vi "MainPanel_20170525.vi"() -> (0 "ErrorOut":errorcluster)   [LabVIEW 2018] (continued)
  # "Cluster data flow is predominantly top to bottom with data being passed using queues.  The Event Structure drives the Main (Consumer) Loop which acts as the Supervisor or dominant loop in this architecture.  In doing so, it handles the functionality of the other loops in your program.  The Consumer Loop processes the 'event' and then if necessary, sends the Master Cluster or a sub-cluster by means of a queue down to the Hardware Loop.  The Hardware loop checks the queued event's data for new information and if there is none, uses the previous iteration's cluster from the Shift Register.  Depending on the mode/event of the Hardware loop, the Hardware Loop may need to update the Master Cluster and does so by pushing the Refresh Panel Queue event which passes the cluster up to the Consumer loop for processing and panel update.  Note that there is a Functional Global inside of the UpdateMasterCluster.vi that is used to maintain a copy of the Master Cluster in memory that can be accessed from anywhere in the software (subVIs included).  This is not always and is often quite unnecessary, but is shown to illustrate a way of passing data between loops without using a Queue.  This use of a FG is quite effective, but must be used with care in that you need to be cautious with where and how often you update the FG; too many writers can cause unpredictable and very challenging code to debug.  The Functional Global exists to allow for any point anywhere in the program and in any loop to grab a copy of your cluster.  This architecture is intended to be a solid starting point for most applications, but you will need to configure and tailor the framework for your specific application and the use of some of the concepts shown herein cannot and should not always be used precisely as shown or at all.\n\nGeneral Rules:\n\n- Don't touch your Hardware anywhere except the HW loop.\n- Try to dedicate loops to very specific tasks to compartmentalize your code as much as possible as this helps with readability and scalability.\n- Any and all periodic updates (logging to disk, graph updates to name two) should occur only in the GUI loop.  Periodic updates of front panel indicators in any other loop will cause unnecessary loop cycles.\n- State changes for the program (ie. Idle, Run, Stop, Error) are handled in the Main Loop only and the panel is updated accordingly. \n- Use the Refresh Panel case in the Main Loop to handle all state changes and Panel GUI configuration tasks (enable/disable controls, visible, colors, alarming, status indicators, etc.).\n- Most loops only run when called by event/queue at the prescribed rate of the software.  Depending on your application, timed or free-wheeling loops could be implemented here if desired, but free-wheeling loops can be inefficient if not carefully implemented.\n- There are a couple of cases such as InitSW that are currently only called upon initialization and never again as shown below and one could argue that they could be outside of the architecture, but if they are called once, they may need to be again, so it is helpful to include them in the overall architecture for potential future use.  An example of this would be InitHW as in the event of a HW failure resulting from poor configuration choices, it would be helpful to be able to call the InitHW case again to reinitialize the HW with new settings."
  n1 = Current VI's Path() -> (path=w82:path)
  n2 = Current VI's Path() -> (path=w88:path)
  n3 = Strip Path(path=w82) -> (stripped path=w81:path)  [unwired: 1 out]
  n4 = Strip Path(path=w88) -> (stripped path=w87:path)  [unwired: 1 out]
  n5 = Strip Path(path=w81) -> (stripped path=w80:path)  [unwired: 1 out]
  n6 = Current VI's Path() -> (path=w98:path)
  n7 = Current VI's Path() -> (path=w90:path)
  n8 = Strip Path(path=w87) -> (stripped path=w86:path)  [unwired: 1 out]
  n9 = Strip Path(path=w98) -> (stripped path=w97:path)  [unwired: 1 out]
  n10 = Strip Path(path=w90) -> (stripped path=w91:path)  [unwired: 1 out]
  n11 = flat-sequence {
    tunnel: [w172] -> w115
    tunnel: errorcluster {"status"=FALSE, "code"=0, "source"=""} ("ErrorIn") -> [w171]
    frame #0 {
      w169 = -1 ("FAM Init 1")
      n12 = shared-variable ".\\Connex_Variables.lvlib\\10Hz_File_Refs"(T45 {"72Co_dset"=0, "84Co_dset"=0, "FileRef"=0} ("10Hz_File_Refs"), error in=w171) -> (error out=w172:errorcluster)
      n13 = shared-variable ".\\Connex_Variables.lvlib\\FAM Init 2"(w169) -> ()  [unwired: 1 in, 1 out]
      n14 = shared-variable ".\\Connex_Variables.lvlib\\FAM Init 1"(w169) -> ()  [unwired: 1 in, 1 out]
      n15 = shared-variable ".\\Connex_Variables.lvlib\\TCP_Status"(TRUE ("TCP_Status")) -> ()  [unwired: 1 in, 1 out]
      n16 = local write "Exit"(FALSE ("Exit")) -> ()
    }
  }
  n17 = Strip Path(path=w97) -> (stripped path=w96:path)  [unwired: 1 out]
  n18 = Strip Path(path=w91) -> (stripped path=w92:path)  [unwired: 1 out]
  n19 = Build Path(base path=w86, name or relative path="NASA\\wtle_young_weather_stn\\WeatherStationMain_20180517.vi") -> (appended path=w84:path)
  n20 = Build Path(base path=w80, name or relative path="NASA\\statmon_2015\\ADAM_health_subpanel_20190329.vi") -> (appended path=w78:path)
  n21 = Obtain Queue(max queue size (-1, unlimited)=100, name (unnamed)="Supervisor", element data type=w165, error in (no error)=w115) -> (queue out=w166:refnum<queue>, error out=w167:errorcluster)  [unwired: 1 in, 1 out]
  n22 = Build Path(base path=w96, name or relative path="Disdrometer\\disdrometer_2020_09_09.vi") -> (appended path=w94:path)
  n23 = Build Path(base path=w92, name or relative path="NASA\\te_2015\\te_20200903.vi") -> (appended path=w89:path)
  n24 = Enqueue Element(queue=w166, element=w165, error in (no error)=w167) -> (queue out=w148:refnum<queue>, error out=w1:errorcluster)  [unwired: 2 out]
  n25 = Open VI Reference(vi path=w78, error in (no error)=w1) -> (vi reference=w74:refnum<vi>, error out=w42:errorcluster)  [unwired: 4 in]
  n26 = Open VI Reference(vi path=w94, error in (no error)=w1) -> (vi reference=w73:refnum<vi>, error out=w57:errorcluster)  [unwired: 4 in]
  n27 = Open VI Reference(vi path=w89, error in (no error)=w1) -> (vi reference=w72:refnum<vi>, error out=w40:errorcluster)  [unwired: 4 in]
  n28 = Open VI Reference(vi path=w84, error in (no error)=w1) -> (vi reference=w16:refnum<vi>, error out=w28:errorcluster)  [unwired: 4 in]
  n29 = invoke on="DisdroPanel" class="SubPnl" method="Insert VI"(error in=w57, "VI Ref"=w73) -> (error out=w54:errorcluster)  [unwired: 2 in, 3 out]
  n30 = invoke on="TE_panel" class="SubPnl" method="Insert VI"(error in=w40, "VI Ref"=w72) -> (error out=w30:errorcluster)  [unwired: 2 in, 3 out]
  n31 = invoke on="Sub Panel - Weather" class="SubPnl" method="Insert VI"(error in=w28, "VI Ref"=w16) -> (error out=w18:errorcluster)  [unwired: 2 in, 3 out]
  n32 = Obtain Queue(max queue size (-1, unlimited)=100, name (unnamed)="Data", element data type=w122, error in (no error)=w1) -> (queue out=w126:refnum<queue>, error out=w124:errorcluster)  [unwired: 1 in, 1 out]
  n33 = Obtain Queue(max queue size (-1, unlimited)=110, name (unnamed)="FP", element data type=w99, error in (no error)=w1) -> (queue out=w102:refnum<queue>, error out=w101:errorcluster)  [unwired: 1 in, 1 out]
  n34 = invoke on="ADAM Health" class="SubPnl" method="Insert VI"(error in=w42, "VI Ref"=w74) -> (error out=w41:errorcluster)  [unwired: 2 in, 3 out]
  n35 = Obtain Queue(max queue size (-1, unlimited)=100, name (unnamed)=w119, element data type=cluster{"HWMd":T25, "Data":variant} {"HWMd"=enum."HW_Init", "Data"=variant}, error in (no error)=w1) -> (queue out=w154:refnum<queue>, error out=w153:errorcluster)  [unwired: 1 in, 1 out]
  n36 = Obtain Queue(max queue size (-1, unlimited)=100, name (unnamed)=w118, element data type=cluster{"HWMd":T25, "Data":variant} {"HWMd"=enum."HW_Init", "Data"=variant}, error in (no error)=w1) -> (queue out=w65:refnum<queue>, error out=w135:errorcluster)  [unwired: 1 in, 1 out]
  n37 = Enqueue Element(queue=w126, element=w122, error in (no error)=w124) -> (queue out=w125:refnum<queue>, error out=w123:errorcluster)  [unwired: 1 in, 1 out]
  n38 = Obtain Queue(max queue size (-1, unlimited)=100, name (unnamed)="10Hz", element data type=cluster{"Enum":T19, "Var":variant} {"Enum"=enum."10Hz_Init", "Var"=variant}) -> (queue out=w14:refnum<queue>, error out=w15:errorcluster)  [unwired: 2 in, 1 out]
  n39 = Obtain Queue(max queue size (-1, unlimited)=1000, name (unnamed)="Tones", element data type=cluster{"Enum":T43, "Data":variant} {"Enum"=enum."Data_Init", "Data"=variant}, error in (no error)=w1) -> (queue out=w149:refnum<queue>, error out=w160:errorcluster)  [unwired: 1 in, 1 out]
  n40 = Obtain Queue(max queue size (-1, unlimited)=100, name (unnamed)="Digi", element data type=w128, error in (no error)=w1) -> (queue out=w132:refnum<queue>, error out=w130:errorcluster)  [unwired: 1 in, 1 out]
  n41 = Obtain Queue(max queue size (-1, unlimited)=100, name (unnamed)="Log", element data type=w4, error in (no error)=w1) -> (queue out=w5:refnum<queue>, error out=w76:errorcluster)  [unwired: 1 in, 1 out]
  n42 = Obtain Queue(max queue size (-1, unlimited)=100, name (unnamed)="TCP", element data type=w7) -> (queue out=w11:refnum<queue>)  [unwired: 2 in, 2 out]
  n43 = Enqueue Element(queue=w102, element=w99, error in (no error)=w101) -> (queue out=w77:refnum<queue>, error out=w100:errorcluster)  [unwired: 1 in, 1 out]
  n44 = Enqueue Element(queue=w5, element=w4, error in (no error)=w76) -> (queue out=w6:refnum<queue>, error out=w12:errorcluster)  [unwired: 1 in, 1 out]
  n45 = Enqueue Element(queue=w11, element=w7) -> (queue out=w2:refnum<queue>, error out=w8:errorcluster)  [unwired: 2 in, 1 out]
  n46 = invoke class="VI" method="Run VI"(reference=w16, error in=w18, "Wait until done"=FALSE ("Wait Until Done"), "Auto Dispose Ref"=FALSE ("Auto Dispose Reference")) -> (error out=w17:errorcluster)  [unwired: 1 in, 4 out]
  n47 = invoke class="VI" method="Run VI"(reference=w74, error in=w41, "Wait until done"=FALSE ("Wait Until Done"), "Auto Dispose Ref"=FALSE ("Auto Dispose Reference")) -> (error out=w43:errorcluster)  [unwired: 1 in, 4 out]
  n48 = invoke class="VI" method="Run VI"(reference=w73, error in=w54, "Wait until done"=FALSE ("Wait Until Done"), "Auto Dispose Ref"=FALSE ("Auto Dispose Reference")) -> (error out=w53:errorcluster)  [unwired: 1 in, 4 out]
  n49 = invoke class="VI" method="Run VI"(reference=w72, error in=w30, "Wait until done"=FALSE ("Wait Until Done"), "Auto Dispose Ref"=FALSE ("Auto Dispose Reference")) -> (error out=w29:errorcluster)  [unwired: 1 in, 4 out]
  n50 = Enqueue Element(queue=w132, element=w128, error in (no error)=w130) -> (queue out=w131:refnum<queue>, error out=w129:errorcluster)  [unwired: 1 in, 1 out]
  n51 = call "NoiseLoop.vi"("error in (no error)"=w123, "Queue in"=w125) -> ("error out"=w147:errorcluster)  [unwired: 9 in]
  n52 = call "LogLoop_HDF5_20190307.vi"("error in"=w12, "Queue in"=w6) -> ("error out"=w109:errorcluster)  [unwired: 9 in]
  n53 = call "Simple TCP - Server_20211123.vi"("error in"=w8, "TCP_Q"=w2) -> ("error out"=w3:errorcluster)  [unwired: 8 in, 1 out]
  n54 = call "DigitalOutput.vi"("error in (no error)"=w129, "Queue in"=w131) -> ("error out"=w120:errorcluster)  [unwired: 9 in]
  n55 = call "10HzLogLoop_HDF5_20210610.vi"("error in"=w15, "queue in"=w14) -> ("error out"=w66:errorcluster)  [unwired: 9 in]
  n56 = while {
    tunnel: w1 -> [w177]
    tunnel: [w175] -> w106
    stop <- w180 stop-if-true
    n57 = call "Elapsed Time"("Time Target (s)"="MemoryPlotRate") -> ("Time has Elapsed"=w179:bool)  [unwired: 11 in, 7 out]
    n58 = Wait Until Next ms Multiple(millisecond multiple=u32 50) -> ()  [unwired: 1 out]
    n59 = case shown="True" w179 {
      tunnel: w177 -> [w181 w184]
      tunnel: [w181 w182] -> w175
      frame False {
      }
      frame True {
        # "When we were using the watchdog to reset Windows,\nwe were checking here. Now that we're only using it to\nnotify WSCR, we're doing it in Log_SSH."
        n60 = constructor class="Process"(error in=w184) -> (reference out=w194:refnum<k24>, error out=w185:errorcluster)  [unwired: 2 in, 1 out]
        n61 = invoke class="Process" method="GetCurrentProcess"(reference=w194, error in=w185) -> (reference out=w192:refnum<k24>, error out=w193:errorcluster, "GetCurrentProcess"=w186:refnum<k24>)  [unwired: 1 in]
        n62 = property class="Process"(reference=w186, error in=w193) -> (reference out=w190:refnum<k24>, error out=w189:errorcluster, "WorkingSet"=w187:i32)
        n63 = Divide(x=w187, y=i64 1024) -> (x/y=→"Memory Used By LV (KB)" →"Memory Used":dbl)
        n64 = Close Reference(reference=w190, error in (no error)=w189) -> (error out=w191:errorcluster)
        n65 = Close Reference(reference=w192, error in (no error)=w191) -> (error out=w182:errorcluster)
      }
    }
    n66 = local read "Exit"() -> (w180:bool)
  }
  n67 = call "TonesLoop_20190705.vi"("WeightOfNewFrequency"=1.0, "error in"=w160, "Queue in"=w149) -> ("error out"=w150:errorcluster)  [unwired: 8 in]
  n68 = while {
    tunnel: w148 -> [w198]
    shift-right: [w197] -> w159
    shift-left: w1 -> [w199]
    stop <- w196 stop-if-true
    n69 = event shown="[7] \"base path\", \"NAS path\", \"ThreshFile\", \"Location\": Value Change" {
      selector: _ -> [_ _ _ _ _ _ _ _ _ _ _ _ _ _]
      dyn-events: _ -> [_ _ _ _ _ _ _ _ _ _ _ _ _ _]
      timeout: 100 -> [_ _ _ _ _ _ _ _ _ _ _ _ _ _]
      tunnel: w199 -> [w204 w208 w221 w227 w229 w233 w241 w249 w257 w260 w265 w269 w273 w277]
      tunnel: w198 -> [_ w215 w216 w222 w230 w234 w242 w250 w258 w262 w266 w270 w274 w279]
      tunnel: [w204 w207 w217 w223 w228 w232 w240 w248 w256 w261 w264 w268 w275 w278] -> w197
      tunnel: [_ w206 _ _ _ _ _ _ _ _ _ _ _ TRUE] -> w196
      event Timeout {
        # "13:24:24.3\n05/31/2018"
        # "Timeout Case is used to update 'heartbeat' clock on the front panel to provide an indication that the software is still running"
        n70 = event-data() -> ()  [unwired: 2 out]
        n71 = Get Date/Time In Seconds() -> (seconds since 1Jan1904=w203:timestamp)
        n72 = Format Date/Time String(time format string (%c)="%H:%M:%S%1u\n%m/%d/%Y", seconds (now)=w203, UTC format=TRUE) -> (date/time string=→"UTC date/time":string)
      }
      event Menu Selection (User) {
        # "This handles a menu selection while the program is running."
        n73 = event-data() -> ("ItemTag"=w209:string)  [unwired: 1 out]
        n74 = Scan From String(input string=w209, error in=w208, default 1=MainQueueElements."Spvsr_InitQ" ("QElmnt")) -> (error out=w205:errorcluster, output 1=w213:T44)  [unwired: 2 in, 2 out]
        n75 = Bundle(cluster=cluster{"QElmnt":T44, "Data":variant} {"QElmnt"=enum."Spvsr_InitQ", "Data"=variant} ("Cluster"), "QElmnt"=w213) -> (w212:cluster{"QElmnt":T44, "Data":variant})  [unwired: 1 in]
        n76 = Enqueue Element(queue=w215, element=w212, error in (no error)=w205) -> (error out=w207:errorcluster)  [unwired: 3 out]
        n77 = Equal?(x=MainQueueElements."Spvsr_Exit" ("QElmnt"), y=w213) -> (x = y?=w206:bool)
      }
      event "Config": Value Change {
        n78 = event-data() -> ()  [unwired: 2 out]
        n79 = Enqueue Element(queue=w216, element=cluster{"QElmnt":T44, "Data":variant} {"QElmnt"=enum."Spvsr_Config", "Data"=variant} ("Cluster"), error in (no error)=w221) -> (error out=w218:errorcluster)  [unwired: 3 out]
        n80 = Enqueue Element(queue=w216, element=cluster{"QElmnt":T44, "Data":variant} {"QElmnt"=enum."Spvsr_FPConfig", "Data"=variant} ("Cluster"), error in (no error)=w218) -> (error out=w217:errorcluster)  [unwired: 3 out]
      }
      event "AutoOffset": Value Change {
        n81 = event-data() -> ()  [unwired: 2 out]
        n82 = Enqueue Element(queue=w222, element=cluster{"QElmnt":T44, "Data":variant} {"QElmnt"=enum."Spvsr_DigitzOffs", "Data"=variant} ("Cluster"), error in (no error)=w227) -> (error out=w224:errorcluster)  [unwired: 3 out]
        n83 = Enqueue Element(queue=w222, element=cluster{"QElmnt":T44, "Data":variant} {"QElmnt"=enum."Spvsr_FPConfig", "Data"=variant} ("Cluster"), error in (no error)=w224) -> (error out=w223:errorcluster)  [unwired: 3 out]
      }
      event "FreqsToRemove", "AvgAvg", "SNR_Thresh", "Width [bins]", "FreqsToRemove 2", "Width 2 [bins]", "SimulateFPGA": Value Change {
        n84 = event-data() -> ()  [unwired: 2 out]
        n85 = Enqueue Element(queue=w230, element=cluster{"QElmnt":T44, "Data":variant} {"QElmnt"=enum."Spvsr_FPConfig", "Data"=variant} ("Cluster"), error in (no error)=w229) -> (error out=w228:errorcluster)  [unwired: 3 out]
      }
      event "MaxTrackRate": Value Change {
        n86 = event-data() -> ()  [unwired: 6 out]
        n87 = for {
          tunnel: cluster{"QElmnt":T44, "Data":variant}[] [{"QElmnt"=enum."Spvsr_FPConfig", "Data"=variant}, {"QElmnt"=enum."Spvsr_TrackRate", "Data"=variant}] ("Cluster") -> [w238] mode=indexing
          tunnel: w234 -> [w237]
          shift-right: [w236] -> w232
          shift-left: w233 -> [w239]
          n88 = Enqueue Element(queue=w237, element=w238, error in (no error)=w239) -> (error out=w236:errorcluster)  [unwired: 3 out]
        }
      }
      event "AutoCenter": Value Change {
        n89 = event-data() -> ()  [unwired: 6 out]
        n90 = for {
          tunnel: cluster{"QElmnt":T44, "Data":variant}[] [{"QElmnt"=enum."Spvsr_FPConfig", "Data"=variant}, {"QElmnt"=enum."Spvsr_AutoCenter", "Data"=variant}] ("Cluster") -> [w246] mode=indexing
          tunnel: w242 -> [w245]
          shift-right: [w244] -> w240
          shift-left: w241 -> [w247]
          n91 = Enqueue Element(queue=w245, element=w246, error in (no error)=w247) -> (error out=w244:errorcluster)  [unwired: 3 out]
        }
      }
      event "base path", "NAS path", "ThreshFile", "Location": Value Change {
        n92 = event-data() -> ()  [unwired: 6 out]
        n93 = for {
          tunnel: cluster{"QElmnt":T44, "Data":variant}[] [{"QElmnt"=enum."Spvsr_FPConfig", "Data"=variant}, {"QElmnt"=enum."Spvsr_RestartWarn", "Data"=variant}] ("Cluster") -> [w254] mode=indexing
          tunnel: w250 -> [w253]
          shift-right: [w252] -> w248
          shift-left: w249 -> [w255]
          n94 = Enqueue Element(queue=w253, element=w254, error in (no error)=w255) -> (error out=w252:errorcluster)  [unwired: 3 out]
        }
      }
      event "Beacon", "Beacon 3": Cursor Move {
        n95 = event-data() -> ()  [unwired: 2 out]
        n96 = Enqueue Element(queue=w258, element=cluster{"QElmnt":T44, "Data":variant} {"QElmnt"=enum."Spvsr_Cursors", "Data"=variant} ("Cluster"), error in (no error)=w257) -> (error out=w256:errorcluster)  [unwired: 3 out]
      }
      event "noise_ctrl", "72GHz_ctrl", "84GHz_ctrl": Value Change {
        n97 = event-data() -> ()  [unwired: 6 out]
        n98 = Enqueue Element(queue=w262, element=cluster{"QElmnt":T44, "Data":variant} {"QElmnt"=enum."FP_AO_ctrl", "Data"=variant} ("Cluster"), error in (no error)=w260) -> (error out=w261:errorcluster)  [unwired: 3 out]
      }
      event "Zoom On Peak", "AutoScale Y Noise", "AutoScale Y Tones": Value Change {
        n99 = event-data() -> ()  [unwired: 2 out]
        n100 = Enqueue Element(queue=w266, element=cluster{"QElmnt":T44, "Data":variant} {"QElmnt"=enum."Spvsr_FPConfig", "Data"=variant} ("Cluster"), error in (no error)=w265) -> (error out=w264:errorcluster)  [unwired: 3 out]
      }
      event Value Change; Key Up {
        n101 = event-data() -> ()  [unwired: 5 out]
        n102 = Enqueue Element(queue=w270, element=cluster{"QElmnt":T44, "Data":variant} {"QElmnt"=enum."Spvsr_AlarmCfg", "Data"=variant} ("Cluster"), error in (no error)=w269) -> (error out=w268:errorcluster)  [unwired: 3 out]
      }
      event "Stop": Value Change {
        n103 = event-data() -> ()  [unwired: 2 out]
        n104 = Enqueue Element(queue=w274, element=cluster{"QElmnt":T44, "Data":variant} {"QElmnt"=enum."Spvsr_Stop", "Data"=variant} ("Cluster"), error in (no error)=w273) -> (error out=w275:errorcluster)  [unwired: 3 out]
      }
      event "Exit": Value Change; Panel Close {
        n105 = event-data() -> ()  [unwired: 2 out]
        n106 = Enqueue Element(queue=w279, element=cluster{"QElmnt":T44, "Data":variant} {"QElmnt"=enum."Spvsr_Exit", "Data"=variant} ("Cluster"), error in (no error)=w277) -> (error out=w278:errorcluster)  [unwired: 3 out]
      }
    }
  }
  n107 = call "AI_Loop.vi"("error in"=w1, "AI_Type"=AI_Type_Enum."AI") -> ("error out"=w121:errorcluster)  [unwired: 9 in]
  n108 = call "AI_Loop.vi"("error in"=w1, "AI_Type"=AI_Type_Enum."TC") -> ("error out"=w112:errorcluster)  [unwired: 9 in]
  n109 = call "AO_Loop.vi"("error"=w1) -> ("error out"=w110:errorcluster)  [unwired: 10 in]
  n110 = while {
    shift-right: [w294] -> w158
    shift-left: w1 -> [w293]
    tunnel: w148 -> [w284]
    shift-right: [w295] -> _
    shift-left: T29 {"Admin"={"Lvl"=enum."Admin", "Pwd"=""}, "RTConfig"={"Arm"=FALSE, "Number"=0.0, "String"=""}, "SMS"={"Enbl?"=FALSE, "Addr"=[]}, "FPGA"={"Target"=enum."1", "Channel"=enum."1", "Ref1"=refnum, "Ref2"=refnum}, "Config"={"UsrCfg"={"Paths"={"CfgFile"=path "", "LogFolder"=path "", "LogFile"=path "", "NAS path"=path "", "ThreshFile"=path "", "RedunFolder"=path ""}, "SampleRate"=0.0}, "FP_User"={"#NoiseSums"=0, "Max_df"=0, "AvgAvg"=FALSE, "#Avg"=0, "AutoCenter"=FALSE, "Inclin"={"Vmin"=0.0, "Vmax"=0.0, "Angle_min"=0.0, "Angle_max"=0.0, "Offset"=0.0, "Pos_Neg"=FALSE}, "1"={"Cal_"={"Fine"=0.0, "Coarse_"=0.0}, "Beac"={"Fine"=0.0, "Coarse_"=0.0}, "Scale"={"Step4"=0.0, "Step5"=0.0, "Step6"=0.0, "Step7"=0.0}, "Offset"=0.0, "Scale_Noise"=0.0, "Scale_Step1"=0.0, "Scale_In_RT"=0.0, "ScaleMeas"=0.0, "FreqsToRemove"=[], "Width"=[], "ScaleMeasEnum"=enum."1", "FilterEnab"=enum."None"}, "2"={"Cal_"={"Fine"=0.0, "Coarse_"=0.0}, "Beac"={"Fine"=0.0, "Coarse_"=0.0}, "Scale"={"Step4"=0.0, "Step5"=0.0, "Step6"=0.0, "Step7"=0.0}, "Offset"=0.0, "Scale_Noise"=0.0, "Scale_Step1"=0.0, "Scale_In_RT"=0.0, "ScaleMeas"=0.0, "FreqsToRemove"=[], "Width"=[], "ScaleMeasEnum"=enum."1", "FilterEnab"=enum."None"}, "3"={"Cal_"={"Fine"=0.0, "Coarse_"=0.0}, "Beac"={"Fine"=0.0, "Coarse_"=0.0}, "Scale"={"Step4"=0.0, "Step5"=0.0, "Step6"=0.0, "Step7"=0.0}, "Offset"=0.0, "Scale_Noise"=0.0, "Scale_Step1"=0.0, "Scale_In_RT"=0.0, "ScaleMeas"=0.0, "FreqsToRemove"=[], "Width"=[], "ScaleMeasEnum"=enum."1", "FilterEnab"=enum."None"}, "4"={"Cal_"={"Fine"=0.0, "Coarse_"=0.0}, "Beac"={"Fine"=0.0, "Coarse_"=0.0}, "Scale"={"Step4"=0.0, "Step5"=0.0, "Step6"=0.0, "Step7"=0.0}, "Offset"=0.0, "Scale_Noise"=0.0, "Scale_Step1"=0.0, "Scale_In_RT"=0.0, "ScaleMeas"=0.0, "FreqsToRemove"=[], "Width"=[], "ScaleMeasEnum"=enum."1", "FilterEnab"=enum."None"}, "Target to Probe"=enum."1", "SNR_Thresh"=0.0, "Paths"={"CfgFile"=path "", "LogFolder"=path "", "LogFile"=path "", "NAS path"=path "", "ThreshFile"=path "", "RedunFolder"=path ""}, "Connex_Location"="", "SimulateFPGA"=FALSE, "Deadband"=0.0}}, "Stat"={"SysState"=enum."Init", "TrackRate"=FALSE, "AutoCentr"=FALSE}, "Alarm"={"TC13"={"Enbl"=FALSE, "ErrsAndWarns"={0.0, 0.0, 0.0, 0.0}}, "AI1"={"Enbl"=FALSE, "ErrsAndWarns"={0.0, 0.0, 0.0, 0.0}}, "AI2"={"Enbl"=FALSE, "ErrsAndWarns"={0.0, 0.0, 0.0, 0.0}}, "AI3"={"Enbl"=FALSE, "ErrsAndWarns"={0.0, 0.0, 0.0, 0.0}}, "AI4"={"Enbl"=FALSE, "ErrsAndWarns"={0.0, 0.0, 0.0, 0.0}}, "AI5"={"Enbl"=FALSE, "ErrsAndWarns"={0.0, 0.0, 0.0, 0.0}}, "AI6"={"Enbl"=FALSE, "ErrsAndWarns"={0.0, 0.0, 0.0, 0.0}}, "AI18"={"Enbl"=FALSE, "ErrsAndWarns"={0.0, 0.0, 0.0, 0.0}}, "AI19"={"Enbl"=FALSE, "ErrsAndWarns"={0.0, 0.0, 0.0, 0.0}}, "TE1"={"Enbl"=FALSE, "ErrsAndWarns"={0.0, 0.0, 0.0, 0.0}}, "TE2"={"Enbl"=FALSE, "ErrsAndWarns"={0.0, 0.0, 0.0, 0.0}}, "TE3"={"Enbl"=FALSE, "ErrsAndWarns"={0.0, 0.0, 0.0, 0.0}}, "ADAM1"={"Enbl"=FALSE, "ErrsAndWarns"={0.0, 0.0, 0.0, 0.0}}, "ADAM2"={"Enbl"=FALSE, "ErrsAndWarns"={0.0, 0.0, 0.0, 0.0}}, "ADAM3"={"Enbl"=FALSE, "ErrsAndWarns"={0.0, 0.0, 0.0, 0.0}}, "ADAM4"={"Enbl"=FALSE, "ErrsAndWarns"={0.0, 0.0, 0.0, 0.0}}, "72CoBeacFreq"={"Enbl"=FALSE, "ErrsAndWarns"={0.0, 0.0, 0.0, 0.0}}, "72CoCalFreq"={"Enbl"=FALSE, "ErrsAndWarns"={0.0, 0.0, 0.0, 0.0}}, "84CoBeacFreq"={"Enbl"=FALSE, "ErrsAndWarns"={0.0, 0.0, 0.0, 0.0}}, "84CoCalFreq"={"Enbl"=FALSE, "ErrsAndWarns"={0.0, 0.0, 0.0, 0.0}}, "72Co_CalTonePwr"={"Enbl"=FALSE, "ErrsAndWarns"={0.0, 0.0, 0.0, 0.0}}, "72X_CalTonePwr"={"Enbl"=FALSE, "ErrsAndWarns"={0.0, 0.0, 0.0, 0.0}}, "84Co_CalTonePwr"={"Enbl"=FALSE, "ErrsAndWarns"={0.0, 0.0, 0.0, 0.0}}, "84X_CalTonePwr"={"Enbl"=FALSE, "ErrsAndWarns"={0.0, 0.0, 0.0, 0.0}}}} ("ClusterIn") -> [w302]
    tunnel: w154 -> [w290]
    tunnel: w149 -> [w289]
    tunnel: w125 -> [w288]
    tunnel: w6 -> [w287]
    tunnel: w77 -> [w286]
    tunnel: w14 -> [w282]
    tunnel: w65 -> [w281]
    i -> [w285]
    stop <- w301 stop-if-true
    # "MasterCluster"
    # "Main \n(Supervisor)\nLoop"
    # "Supervisor Loop"
    n111 = call "PushToErrorHandler.vi"("ErrorIn"=w293, "ErrorLocation"="Supervisor") -> ("ErrorOut"=w292:errorcluster)  [unwired: 5 in]
    n112 = Get Queue Status(queue=w284) -> (# elements in queue=→"SPVSR_Queue":i32)  [unwired: 2 in, 7 out]
    n113 = Dequeue Element(queue=w284, error in (no error)=w292) -> (queue out=w300:refnum<queue>, element=w298:cluster{"QElmnt":T44, "Data":variant}, error out=w299:errorcluster)  [unwired: 2 out]
    n114 = Unbundle(w298) -> ("QElmnt"=w297:T44, "Data"=w296:variant)
    n115 = case shown="\"Spvsr_ChkTime\"" w297 {
      tunnel: w299 -> [w313 w323 w404 w413 w447 w453 w481 w504 w511 w523 w596 w659 w687 w706 w741 w765 w831 w835 w837 w857 w890 w892]
      tunnel: [w312 w348 w398 w412 w445 w459 w478 w506 w508 w527 w591 w613 w689 w714 w732 w764 w830 w834 w838 w842 w888 w896] -> w295
      tunnel: w302 -> [w312 w349 w398 w415 w445 w460 w478 w507 w508 w528 w597 w603 w686 w713 w732 w764 w829 w833 w838 w854 w888 w896]
      tunnel: [_ _ _ _ _ _ _ _ _ _ _ _ _ _ _ _ _ _ _ _ _ TRUE] -> w301
      tunnel: [w311 w350 w404 w409 w436 w454 w479 w501 w510 w530 w593 w658 w683 w706 w727 w765 w831 w835 w837 w841 w889 w893] -> w294
      tunnel: w300 -> [w314 _ _ _ _ w450 _ w502 _ w524 _ _ _ _ _ _ _ _ _ w864 _ _]
      tunnel: w296 -> [_ _ _ w414 _ _ _ _ w509 w525 _ _ _ _ _ _ _ _ _ _ _ _]
      tunnel: w290 -> [_ _ _ _ _ _ _ _ _ w529 _ _ _ _ _ _ _ _ _ _ _ _]
      tunnel: w289 -> [_ _ _ _ _ _ _ _ _ _ _ w657 _ _ _ _ _ _ _ _ _ w895]
      tunnel: w288 -> [_ _ _ _ _ _ _ _ _ _ _ w652 _ _ _ _ _ _ _ _ _ w894]
      tunnel: w287 -> [_ _ _ _ _ _ _ _ _ _ _ w629 w682 _ w726 _ _ _ _ _ _ _]
      tunnel: w286 -> [_ _ _ _ _ _ _ _ _ _ _ _ _ _ _ _ _ _ _ _ _ _]
      tunnel: w282 -> [_ _ _ _ _ _ _ _ _ _ _ _ _ _ _ _ _ _ _ _ _ w891]
      tunnel: w281 -> [_ _ _ _ _ _ _ _ _ _ _ _ _ _ _ _ _ _ _ _ _ _]
      frame "Spvsr_InitQ" {
        # "This case is called upon launch and calls all cases necessary to initialize the application."
        n116 = Build Array(cluster{"QElmnt":T44, "Data":variant} {"QElmnt"=enum."Spvsr_InitSW", "Data"=variant} ("Cluster"), cluster{"QElmnt":T44, "Data":variant} {"QElmnt"=enum."Spvsr_InitCtrls", "Data"=variant} ("Cluster"), cluster{"QElmnt":T44, "Data":variant} {"QElmnt"=enum."Spvsr_FPConfig", "Data"=variant} ("Cluster"), cluster{"QElmnt":T44, "Data":variant} {"QElmnt"=enum."Spvsr_AlarmCfg", "Data"=variant} ("Cluster"), cluster{"QElmnt":T44, "Data":variant} {"QElmnt"=enum."Spvsr_StrtHWLp", "Data"=variant} ("Cluster"), cluster{"QElmnt":T44, "Data":variant} {"QElmnt"=enum."Spvsr_RfrshPnl", "Data"=variant} ("Cluster"), cluster{"QElmnt":T44, "Data":variant} {"QElmnt"=enum."Spvsr_ChkTime", "Data"=variant} ("Cluster")) -> (w305:cluster{"QElmnt":T44, "Data":variant}[])
        n117 = for {
          tunnel: w314 -> [w318]
          tunnel: w305 -> [w315] mode=indexing
          shift-right: [w316] -> w311
          shift-left: w313 -> [w317]
          n118 = Enqueue Element(queue=w318, element=w315, error in (no error)=w317) -> (error out=w316:errorcluster)  [unwired: 1 in, 2 out]
        }
      }
      frame "Spvsr_InitSW" {
        # "Reset\nWatchdog"
        # "These files are updated in the tones (Data) loop"
        # "This case is used to initialize the startup conditions for your software."
        n119 = call "MountNAS.vi"("error in"=w323) -> ("error out"=w322:errorcluster)  [unwired: 10 in]
        n120 = call "InitSupervisorCluster.vi"("error in (no error)"=w322, "ClusterIn in"=w349) -> ("error out"=w326:errorcluster, "ClusterIn out"=w353:T29)  [unwired: 8 in]
        n121 = call "PushToErrorHandler.vi"("ErrorIn"=w326, "ErrorLocation"="InitClust") -> ("ErrorOut"=w325:errorcluster)  [unwired: 5 in]
        n122 = call "ReadConfigFile.vi"("ErrorIn"=w325, "ClusterIn"=w353) -> ("ErrorOut"=w330:errorcluster, "dup path"=w333:path, "ClusterOut"=w332:T29)  [unwired: 1 in, 6 out]
        n123 = call "ReadThreshFile_20200519.vi"("MainClust"=w332) -> ("ErrorOut"=w329:errorcluster, "dup path"=w328:path, "MainClustOut"=w331:T29)  [unwired: 8 in]
        n124 = case shown="Error" w330 {
          tunnel: w333 -> [_ w365]
          frame No Error {
          }
          frame Error {
            # "This triggers the\n\"exit\" event."
            n125 = property on="Exit" class="Bool (strict)"("Val(Sgnl)"=TRUE ("Value (Signaling)")) -> ()  [unwired: 2 in, 2 out]
            n126 = Path To String(path=w365) -> (string=w364:string)
            n127 = Concatenate Strings("Unfortunately, there is a problem with your configuration file.\nThis software will not run properly with the configuration file you have. \n\nYou can likely fix the problem by simply renaming your existing file and reconfiguring the system. \n\nThe file is found at:", w364, "\r\n", "For help with this, please contact Epimedia at 1.888.374.6334\n\nError 1108 " ("string")) -> (w361:string)
            n128 = One Button Dialog(message=w361) -> ()  [unwired: 1 in, 1 out]
          }
        }
        n129 = case shown="Error" w329 {
          tunnel: w328 -> [_ w358]
          frame No Error {
          }
          frame Error {
            n130 = Path To String(path=w358) -> (string=w357:string)
            n131 = Concatenate Strings("Unfortunately, there is a problem with your thresholds file.\nThis software will not run properly with the thresholds file you have. \n\nThe file is expected at:", w357, "\r\n", "For help with this, please contact Epimedia at 1.888.374.6334\n\nError 1109 " ("string")) -> (w354:string)
            n132 = One Button Dialog(message=w354) -> ()  [unwired: 1 in, 1 out]
          }
        }
        n133 = call <vilib>:"Clear Errors.vi"("error in (no error)"=w329) -> ("error out"=w327:errorcluster)  [unwired: 5 in, 1 out]
        n134 = call "InitFreqFiles.vi"("error in"=w327, "FileName"="72.txt") -> ("error out"=w343:errorcluster, "value"=w334:dbl)  [unwired: 7 in, 1 out]
        n135 = Subtract(x=w334, y=2500.0 ("x")) -> (x-y=w335:dbl)
        n136 = call "InitFreqFiles.vi"("error in"=w343, "FileName"="84.txt") -> ("error out"=w320:errorcluster, "value"=w342:dbl)  [unwired: 7 in, 1 out]
        n137 = Bundle By Name(cluster=T11 {"Fine"=0.0, "Coarse_"=0.0} ("72 Beac"), "Coarse_"=w335) -> (w341:T11)
        n138 = Subtract(x=w342, y=2500.0 ("x")) -> (x-y=w338:dbl)
        n139 = Bundle By Name(cluster=T11 {"Fine"=0.0, "Coarse_"=0.0} ("72 Beac"), "Coarse_"=w338) -> (w340:T11)
        n140 = call "Watchdog_Functional_Global.vi"("Watchdog"=WatchdogTimer_Enum."ResetAll", "error in"=w320) -> ("error out"=w319:errorcluster)  [unwired: 7 in, 2 out]
        n141 = Bundle By Name(cluster=w331, "Config.FP_User.Max_df"=u32 1, "Config.FP_User.1.Beac"=w341, "Config.FP_User.2.Beac"=w341, "Config.FP_User.3.Beac"=w340, "Config.FP_User.4.Beac"=w340) -> (w348:T29)
        n142 = Not(x=TRUE ("Visible")) -> (.not. x?=w351:bool)
        n143 = property on="Stop" class="Bool"(error in=w319, "Visible"=w351) -> (error out=w350:errorcluster)  [unwired: 1 in, 1 out]
      }
      frame "Spvsr_InitCtrls" {
        w397 = TRUE ("72GHz_ctrl")
        # "Distinct \"Redundant Folder\" no longer used."
        # "# of sums of noise floor to be recorded is no longer user-configurable."
        # "# Averages in FPGA no longer user configurable. Always 150."
        # "Cal shift is recorded as a negative value and must be corrected here for display.\nBeac shift is changed to positive before it is recorded."
        # "Auto Center must be off at startup. FFT is nonsense at startup. Auto Center will jump to 0 and never move."
        # "Initalize controls with values from config file."
        n144 = Unbundle By Name(w398) -> ("Config.FP_User.AvgAvg"=w403:bool, "Config.FP_User.1.Cal_"=w402:T11, "Config.FP_User.1.Beac"=w401:T11, "Config.FP_User.1.FilterEnab"=w385:T5, "Config.FP_User.1.ScaleMeas"=w394:fxp<+/-,16,1>, "Config.FP_User.1.Scale_Step1"=w393:fxp<+/-,17,17>, "Config.FP_User.1.Scale"=w392:T4, "Config.FP_User.1.Offset"=w374:fxp<+/-,16,16>, "Config.FP_User.2.Offset"=w373:fxp<+/-,16,16>, "Config.FP_User.3.Offset"=w372:fxp<+/-,16,16>, "Config.FP_User.4.Offset"=w371:fxp<+/-,16,16>, "Config.FP_User.1.FreqsToRemove"=w400:i32[], "Config.FP_User.Target to Probe"=w399:T16, "Config.FP_User.3.FreqsToRemove"=w376:i32[], "Config.FP_User.3.Width"=w375:i32[], "Config.FP_User.SNR_Thresh"=w377:dbl, "Config.FP_User.Paths.LogFolder"=w386:path, "Config.FP_User.Paths.NAS path"=w387:path, "Config.FP_User.Paths.ThreshFile"=w388:path, "Config.FP_User.Connex_Location"=w389:string, "Config.FP_User.Max_df"=w390:u32, "Config.FP_User.1.Width"=w384:i32[], "Config.FP_User.Inclin"=w381:T7, "Alarm"=w378:T13, "Config.FP_User.Deadband"=w367:dbl)  [unwired: 5 out]
        n145 = local write "FilterEnable"(w385) -> ()
        n146 = local write "AvgAvg"(w403) -> ()
        n147 = local write "AutoCenter"(FALSE ("AutoCenter")) -> ()
        n148 = local write "Deadband"(w367) -> ()
        n149 = local write "AlarmSettings"(w378) -> ()
        n150 = local write "Width [bins]"(w384) -> ()
        n151 = Bundle By Name(cluster=T3 {"Measure"=0.050018310546875, "Step1"=2.0, "Scale"={"Step4"=3.0, "Step5"=1.0, "Step6"=1.0, "Step7"=1.0}} ("Scale"), "Measure"=w394, "Step1"=w393, "Scale"=w392) -> (w391:T3)
        n152 = local write "FreqsToRemove 2"(w376) -> ()
        n153 = local write "FreqsToRemove"(w400) -> ()
        n154 = local write "Target to Probe"(w399) -> ()
        n155 = local write "Width 2 [bins]"(w375) -> ()
        n156 = local write "SNR_Thresh"(w377) -> ()
        n157 = local write "base path"(w386) -> ()
        n158 = local write "NAS path"(w387) -> ()
        n159 = local write "ThreshFile"(w388) -> ()
        n160 = local write "Location"(w389) -> ()
        n161 = local write "MaxTrackRate"(w390) -> ()
        n162 = local write "Inclin"(w381) -> ()
        n163 = local write "Scale"(w391) -> ()
        n164 = local write "Digitizer Offset 72 Co"(w374) -> ()
        n165 = local write "Digitizer Offset 72 X"(w373) -> ()
        n166 = local write "Digitizer Offset 84 Co"(w372) -> ()
        n167 = local write "Digitizer Offset 84 x"(w371) -> ()
        n168 = Negate(x=w402) -> (-x=w380:T11)
        n169 = local write "RightSideTab"(T1."Power Hist" ("RightSideTab")) -> ()
        n170 = local write "LeftSideTab"(T9."Weather" ("LeftSideTab")) -> ()
        n171 = local write "Shift Cal"(w380) -> ()
        n172 = local write "Shift Beac"(w401) -> ()
        n173 = Unbundle By Name(w398) -> ("Config.FP_User.3.Cal_"=w383:T11, "Config.FP_User.3.Beac"=w382:T11)
        n174 = local write "SimulateFPGA"(FALSE ("SimulateFPGA")) -> ()
        n175 = local write "84GHz_ctrl"(w397) -> ()
        n176 = local write "72GHz_ctrl"(w397) -> ()
        n177 = Negate(x=w383) -> (-x=w379:T11)
        n178 = local write "Shift Cal 3"(w379) -> ()
        n179 = local write "Shift Beac 3"(w382) -> ()
      }
      frame "Spvsr_RfrshPnl" {
        # "The User level can be used here to configure controls/indicators depending on user privileges."
        # "Use this case to handle all VI panel updates corresponding to program state changes such as enabling/disabling controls based on system states such as HW Mode."
        n180 = call "CheckVariantForClusterUpdate_MainLoop.vi"("ErrorIn"=w413, "VariantIn"=w414, "ClusterIn"=w415) -> ("ErrorOut"=w407:errorcluster, "ClusterOut"=w412:T29)  [unwired: 7 in]
        n181 = Unbundle By Name(w412) -> ("Stat.SysState"=w411:T42, "Admin.Lvl"=w410:T31)
        n182 = case shown="\"Idle\"" w411 {
          tunnel: [T48."Disabled and Grayed Out" ("Disabled") T48."Enabled" ("Disabled") T48."Disabled and Grayed Out" ("Disabled") T48."Disabled and Grayed Out" ("Disabled") T48."Disabled and Grayed Out" ("Disabled") T48."Disabled and Grayed Out" ("Disabled")] -> w408
          tunnel: [T48."Disabled and Grayed Out" ("Disabled") T48."Disabled and Grayed Out" ("Disabled") T48."Disabled and Grayed Out" ("Disabled") T48."Enabled" ("Disabled") T48."Disabled and Grayed Out" ("Disabled") T48."Disabled and Grayed Out" ("Disabled")] -> _
          tunnel: [FALSE FALSE FALSE FALSE TRUE FALSE] -> w406
          frame "Init" {
          }
          frame "Idle" {
          }
          frame "Running" {
          }
          frame "System Fault" {
          }
          frame "System Error" {
          }
          frame "Exit" {
          }
        }
        n183 = case shown="\"Operator\"" w410 {
          frame "Admin", Default {
          }
          frame "Operator" {
          }
        }
        n184 = property on="SysErr" class="Str"(error in=w407, "Visible"=w406) -> (error out=w405:errorcluster)  [unwired: 1 in, 1 out]
        n185 = property on="Stop" class="Bool"(error in=w405, "DisabledEnum"=w408) -> (error out=w409:errorcluster)  [unwired: 1 in, 1 out]
      }
      frame "Spvsr_Cursors" {
        n186 = control-ref of="Beacon"() -> (w449:refnum<vi>)
        n187 = control-ref of="Beacon 2"() -> (w442:refnum<vi>)
        n188 = property class="WFGraph (strict)"(reference=w449, error in=w447) -> (error out=w448:errorcluster, "CrsrList"=w443:T50, "Active Cursor"=w444:u32, "Cursor.Cursor X"=w446:dbl)  [unwired: 1 out]
        n189 = property class="WFGraph (strict)"(reference=w442, error in=w448, "CrsrList"=w443, "Active Cursor"=w444, "Cursor.Cursor X"=w446) -> (error out=w437:errorcluster)  [unwired: 1 out]
        n190 = control-ref of="Beacon 3"() -> (w435:refnum<vi>)
        n191 = control-ref of="Beacon 4"() -> (w434:refnum<vi>)
        n192 = property class="WFGraph (strict)"(reference=w435, error in=w437) -> (error out=w438:errorcluster, "CrsrList"=w441:T50, "Active Cursor"=w440:u32, "Cursor.Cursor X"=w439:dbl)  [unwired: 1 out]
        n193 = property class="WFGraph (strict)"(reference=w434, error in=w438, "CrsrList"=w441, "Active Cursor"=w440, "Cursor.Cursor X"=w439) -> (error out=w436:errorcluster)  [unwired: 1 out]
      }
      frame "Spvsr_Admin" {
        # "This case handles the Admin/Operator menu selection and you can use this to configure your software behavior depending on User Level.  The appropriate place to do this is to read the User Level in the Refresh Panel and set the behavior and appearance of your controls/indicators appropriately."
        n194 = Enqueue Element(queue=w450, element=cluster{"QElmnt":T44, "Data":variant} {"QElmnt"=enum."Spvsr_RfrshPnl", "Data"=variant} ("Cluster"), error in (no error)=w453) -> (error out=w452:errorcluster)  [unwired: 3 out]
        n195 = Unbundle By Name(w460) -> ("Admin.Lvl"=w461:T31, "Admin.Pwd"=w458:string)
        n196 = case shown="\"Operator\", Default" w461 {
          tunnel: w452 -> [w463 w470]
          tunnel: [w463 w466] -> w455
          tunnel: [UserLevelEnum."Operator" ("UserLevel") w467] -> w457
          tunnel: w458 -> [_ w464]
          frame "Admin" {
          }
          frame "Operator", Default {
            n197 = call "AdminLogon.vi"("ErrorIn"=w470, "Password"=w464) -> ("ErrorOut"=w466:errorcluster, "Successful?"=w465:bool)  [unwired: 8 out]
            n198 = Select(t=UserLevelEnum."Admin" ("UserLevel"), s=w465, f=UserLevelEnum."Operator" ("UserLevel")) -> (s? t:f=w467:T31)
          }
        }
        n199 = Current VI's Menubar() -> (w456:refnum<k9>)
        n200 = call "MenuConfiguration.vi"("UserLevel"=w457, "ErrorIn"=w455, "MenuRef"=w456) -> ("ErrorOut"=w454:errorcluster)  [unwired: 8 out]
        n201 = Bundle By Name(cluster=w460, "Admin.Lvl"=w457) -> (w459:T29)
      }
      frame "Spvsr_StrtHWLp" {
        # "If there is a problem with the thresholds file,\ndo not start the AI loop."
        # "Starts the HW Loop and this should only be called once all Main Loop and Software Initialization has occurred to ensure that the HW Loop has the newest data to operate on."
        n202 = Build Array(cluster{"HWMd":T25, "Data":variant} {"HWMd"=enum."HW_Init", "Data"=variant}) -> (w480:cluster{"HWMd":T25, "Data":variant}[])
        n203 = call "Init_All_FPGAs.vi"("error in (no error)"=w481, "Array"=w480) -> ("error out"=w475:errorcluster)  [unwired: 9 in]
        n204 = call "PushToErrorHandler.vi"("ErrorIn"=w475, "ErrorLocation"="InitFPGAs") -> ("ErrorOut"=w472:errorcluster)  [unwired: 5 in]
        n205 = Unbundle By Name(w478) -> ("Alarm"=w473:T13, "Config.FP_User.Inclin"=w476:T7)
        n206 = Bundle(cluster=cluster{"Alarm":T13, "Inclin":T7} {"Alarm"={"TC13"={"Enbl"=FALSE, "ErrsAndWarns"={0.0, 0.0, 0.0, 0.0}}, "AI1"={"Enbl"=FALSE, "ErrsAndWarns"={0.0, 0.0, 0.0, 0.0}}, "AI2"={"Enbl"=FALSE, "ErrsAndWarns"={0.0, 0.0, 0.0, 0.0}}, "AI3"={"Enbl"=FALSE, "ErrsAndWarns"={0.0, 0.0, 0.0, 0.0}}, "AI4"={"Enbl"=FALSE, "ErrsAndWarns"={0.0, 0.0, 0.0, 0.0}}, "AI5"={"Enbl"=FALSE, "ErrsAndWarns"={0.0, 0.0, 0.0, 0.0}}, "AI6"={"Enbl"=FALSE, "ErrsAndWarns"={0.0, 0.0, 0.0, 0.0}}, "AI18"={"Enbl"=FALSE, "ErrsAndWarns"={0.0, 0.0, 0.0, 0.0}}, "AI19"={"Enbl"=FALSE, "ErrsAndWarns"={0.0, 0.0, 0.0, 0.0}}, "TE1"={"Enbl"=FALSE, "ErrsAndWarns"={0.0, 0.0, 0.0, 0.0}}, "TE2"={"Enbl"=FALSE, "ErrsAndWarns"={0.0, 0.0, 0.0, 0.0}}, "TE3"={"Enbl"=FALSE, "ErrsAndWarns"={0.0, 0.0, 0.0, 0.0}}, "ADAM1"={"Enbl"=FALSE, "ErrsAndWarns"={0.0, 0.0, 0.0, 0.0}}, "ADAM2"={"Enbl"=FALSE, "ErrsAndWarns"={0.0, 0.0, 0.0, 0.0}}, "ADAM3"={"Enbl"=FALSE, "ErrsAndWarns"={0.0, 0.0, 0.0, 0.0}}, "ADAM4"={"Enbl"=FALSE, "ErrsAndWarns"={0.0, 0.0, 0.0, 0.0}}, "72CoBeacFreq"={"Enbl"=FALSE, "ErrsAndWarns"={0.0, 0.0, 0.0, 0.0}}, "72CoCalFreq"={"Enbl"=FALSE, "ErrsAndWarns"={0.0, 0.0, 0.0, 0.0}}, "84CoBeacFreq"={"Enbl"=FALSE, "ErrsAndWarns"={0.0, 0.0, 0.0, 0.0}}, "84CoCalFreq"={"Enbl"=FALSE, "ErrsAndWarns"={0.0, 0.0, 0.0, 0.0}}, "72Co_CalTonePwr"={"Enbl"=FALSE, "ErrsAndWarns"={0.0, 0.0, 0.0, 0.0}}, "72X_CalTonePwr"={"Enbl"=FALSE, "ErrsAndWarns"={0.0, 0.0, 0.0, 0.0}}, "84Co_CalTonePwr"={"Enbl"=FALSE, "ErrsAndWarns"={0.0, 0.0, 0.0, 0.0}}, "84X_CalTonePwr"={"Enbl"=FALSE, "ErrsAndWarns"={0.0, 0.0, 0.0, 0.0}}}, "Inclin"={"Vmin"=0.0, "Vmax"=0.0, "Angle_min"=0.0, "Angle_max"=0.0, "Offset"=0.0, "Pos_Neg"=FALSE}}, "Alarm"=w473, "Inclin"=w476) -> (w477:cluster{"Alarm":T13, "Inclin":T7})
        n207 = case shown="No Error" w472 {
          tunnel: [w484 errorcluster {"status"=FALSE, "code"=0, "source"=""} ("error out")] -> w479
          tunnel: w477 -> [w483 _]
          frame No Error {
            n208 = To Variant(anything=w483) -> (Variant=w486:variant)
            n209 = Bundle By Name(cluster=cluster{"Enum":T49, "Var":variant} {"Enum"=enum."AI_Init", "Var"=variant}, "Var"=w486) -> (w487:cluster{"Enum":T49, "Var":variant})
            n210 = Build Array("AI" ("name (unnamed)"), "TC" ("name (unnamed)")) -> (w485:string[])
            n211 = for {
              tunnel: w487 -> [w493]
              tunnel: w485 -> [w492] mode=indexing
              shift-right: [w491] -> w484
              shift-left: _ -> [w494]
              n212 = Obtain Queue(max queue size (-1, unlimited)=100, name (unnamed)=w492, element data type=w493, error in (no error)=w494) -> (queue out=w499:refnum<queue>, error out=w497:errorcluster)  [unwired: 1 in, 1 out]
              n213 = Enqueue Element(queue=w499, element=w493, error in (no error)=w497) -> (queue out=w495:refnum<queue>, error out=w496:errorcluster)  [unwired: 1 in, 1 out]
              n214 = Release Queue(queue=w495, error in (no error)=w496) -> (error out=w491:errorcluster)  [unwired: 1 in, 2 out]
            }
          }
          frame Error {
          }
        }
      }
      frame "Spvsr_Stop" {
        # "The Stop case would stop the execution of a currently running test.  The System State is updated and Refresh Panel is called so that the front panel controls can be configured for this state."
        n215 = Enqueue Element(queue=w502, element=cluster{"QElmnt":T44, "Data":variant} {"QElmnt"=enum."Spvsr_RfrshPnl", "Data"=variant} ("Cluster"), error in (no error)=w504) -> (error out=w501:errorcluster)  [unwired: 3 out]
        n216 = Bundle By Name(cluster=w507, "Stat.SysState"=SystemStateEnum."Idle") -> (w506:T29)
      }
      frame "Spvsr_NewData" {
        n217 = Variant To Data(error in=w511, type=T32 {"Arm"=FALSE, "Number"=0.0, "String"=""} ("RTConfig"), Variant=w509) -> (data=w514:T32, error out=w510:errorcluster)
        n218 = Unbundle By Name(w508) -> ("RTConfig"=w513:T32)
        n219 = Equal?(x=w513, y=w514) -> ()  [unwired: 1 out]
      }
      frame "Spvsr_Error" {
        # "The Error Handler case can be called from anywhere in the software and is called using the PushToErrorHandler.vi.  This allows for the software to handle errors in one spot in the software while allowing the Main Loop to push a new state to the HW and other loops.  Note that for the user defined error code 5000, conditions (HW Disabled) are set, an event is sent down to instantly reconfigure the system and THEN the message dialog box can be popped up for the user.  In some cases, you may not want to popup a dialog box (as shown below for 5000), but merely clear an error and reset or pause hardware. \n\nIt is an impossible task to define exactly how all software should behave with respect to handling error, but the most important thing is that as a developer, you must consider all possible sources of error and to ensure that your software responds appropriately.  The PushToErrorHandler.vi should be used frequently to ensure that you trap all errors as if there is a potential for an error to occur, you should consider how your software will behave when that error occurs and how you need/want to present this error to the user."
        n220 = Enqueue Element(queue=w524, element=cluster{"QElmnt":T44, "Data":variant} {"QElmnt"=enum."Spvsr_RfrshPnl", "Data"=variant} ("Cluster"), error in (no error)=w523) -> (error out=w522:errorcluster)  [unwired: 3 out]
        n221 = Variant To Data(error in=w522, type=w522, Variant=w525) -> (data=w526:errorcluster, error out=w518:errorcluster)
        n222 = Unbundle By Name(w526) -> ("code"=w519:i32)
        n223 = call "CheckForExistingErrorDialog.vi"("ErrorIn"=w518, "ErrorCodeIn"=w519) -> ("ErrorOut"=w516:errorcluster, "NoWndwFnd"=w515:bool, "ErrorCodeOut"=w517:i32)  [unwired: 7 in]
        n224 = call "PushToErrorHandler.vi"("ErrorIn"=w516, "ErrorLocation"="Error Handler") -> ("ErrorOut"=w531:errorcluster)  [unwired: 5 in]
        n225 = case shown="True" w515 {
          tunnel: w531 -> [w532 w540]
          tunnel: [w532 w539] -> w530
          tunnel: w529 -> [_ w538]
          tunnel: w528 -> [w533 w537]
          tunnel: [w533 w536] -> w527
          tunnel: w526 -> [_ w535]
          tunnel: w517 -> [_ w534]
          frame False {
          }
          frame True {
            n226 = case shown="-8998" w534 {
              tunnel: [w548 w557 w559 w566 w570 w577 w586] -> w539
              tunnel: w537 -> [w544 w553 w560 w565 w572 w582 w584]
              tunnel: [w543 w552 w561 w565 w573 w576 w584] -> w536
              tunnel: w540 -> [w549 w558 w559 w564 w570 w578 w587]
              tunnel: w535 -> [w547 w556 _ w567 _ w579 w588]
              tunnel: w538 -> [_ _ _ _ _ _ _]
              frame Default {
                # "-1 dictates that the message box does NOT time out"
                # "Default Error Case handles all error codes undefined by this structure."
                n227 = Bundle By Name(cluster=w544, "Stat.SysState"=SystemStateEnum."System Fault") -> (w543:T29)
                n228 = Unbundle By Name(w543) -> ("SMS"=w542:T33)
